vi "ClassClearMutationHistory.vi"() -> ()   [LabVIEW 2020]
uses:
  <vilib>/Utility/EditLVLibs/Edit LVLibs.lvlib
panel:
  out "Path":path
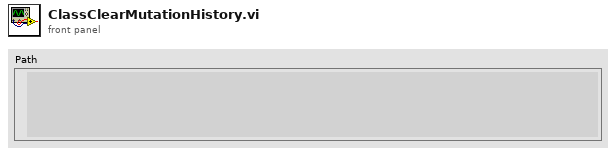
[diagram p1: front panel]
types:
  T1 = typedef "Edit LVLibs.lvlib/Mutation History.ctl" = T2[]
  T2 = typedef "Edit LVLibs.lvlib/Mutation Record.ctl" = cluster{"Library Version":T3, "Old Name Index":u8, "Class Default Data":variant, "Cluster Order Map":u32[], "Parent Name":string, "Parent Path":path, "LabVIEW Version":u32, "User Comments":string, "Mutation Flags":u8, "Parent Old Name Index":u8, "Parent Levels Added":u16, "Parent Levels Removed":u16}
  T3 = typedef "Edit LVLibs.lvlib/LibVersion.ctl" = cluster{"Major":u16, "Minor":u16, "Fix":u16, "Build":u16}
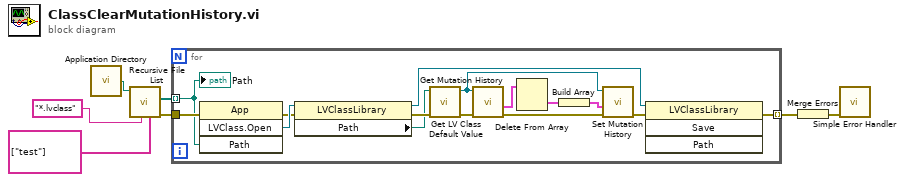
[diagram p0: block diagram]
diagram:
  n1 = call <vilib>:"Application Directory.vi"() -> ("Application Directory"=w7:path)
  n2 = call <vilib>:"Recursive File List.vi"("Folders to Exclude"=string[] ["test"], "pattern"="*.lvclass", "Folder Path"=w7) -> ("error out"=w5:errorcluster, "All Files in Dir"=w4:path[])  [unwired: 4 in, 3 out]
  n3 = for {
    tunnel: w5 -> [w18]
    tunnel: w4 -> [w13] mode=indexing
    tunnel: [w10] -> w3 mode=indexing
    n4 = invoke class="App" method="LVClass.Open"(error in=w18, "Path"=w13) -> (error out=w16:errorcluster, "LVClass.Open"=w17:refnum<vi>)  [unwired: 2 in, 2 out]
    n5 = property class="LVClassLibrary"(reference=w17, error in=w16) -> (reference out=w11:refnum<vi>, error out=w15:errorcluster, "Path"=w14:path)
    n6 = call <vilib>:"Get LV Class Default Value.vi"("error in (no error)"=w15, "class path"=w14) -> ("error out"=w22:errorcluster, "object"=w19:refnum<class>)  [unwired: 8 in]
    n7 = call <vilib>:"Get Mutation History.vi"("error in"=w22, "Input object"=w19) -> ("error out"=w20:errorcluster, "Mutation History"=w21:T1)  [unwired: 6 in]
    n8 = Delete From Array(array=w21) -> (deleted portion=w9:T2)  [unwired: 2 in, 1 out]
    n9 = Build Array(w9) -> (w8:T2[])
    n10 = call <vilib>:"Set Mutation History.vi"("error in"=w20, "Mutation History"=w8, "Input object"=w19) -> ("error out"=w12:errorcluster)  [unwired: 8 in]
    n11 = invoke class="LVClassLibrary" method="Save"(reference=w11, error in=w12) -> (error out=w10:errorcluster)  [unwired: 2 in, 3 out]
    "Path" <- w13
  }
  n12 = Merge Errors(w3) -> (w2:errorcluster)
  n13 = call <vilib>:"Simple Error Handler.vi"("error in (no error)"=w2) -> ()  [unwired: 4 in, 5 out]
